vi "Array Edit.vi"(9 "Number of Points":i32, 11 "Y-values":dbl[](array[numeric])) -> (3 "Editted Y Values":dbl[](array[numeric]))   [LabVIEW 2014]
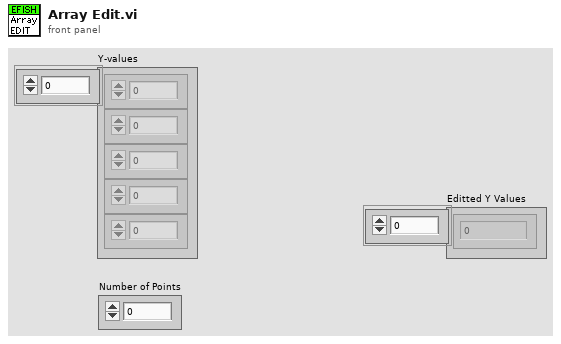
[diagram p1: front panel]
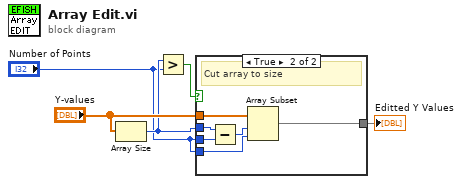
[diagram p0: block diagram]
diagram:
  n1 = Array Size(array="Y-values") -> (size(s)=w3:i32)
  n2 = Greater?(x=w3, y="Number of Points") -> (0:w5:bool)
  n3 = case shown="True" w5 {
    tunnel: "Y-values" -> [w6 w12]
    tunnel: "Number of Points" -> [_ w11]
    tunnel: w3 -> [_ w10]
    tunnel: "Number of Points" -> [_ w9]
    tunnel: [w6 w7] -> w2
    frame False {
      # "no need to edit"
    }
    frame True {
      # "Cut array to size"
      n4 = Subtract(x=w10, y=w9) -> (x-y=w8:i32)
      n5 = Array Subset(array=w12, index=w8, length=w11) -> (w7:dbl[])
    }
  }
  "Editted Y Values" <- w2
